vi "value to ring (portSpeed).vi"(11 "value":string) -> (3 "portSpeed":u32)   [LabVIEW 2020, in "AIM ARINC 664 Import.lvlib"]
uses:
  AIM ARINC 664 Import.lvlib
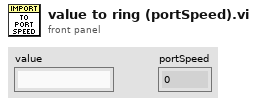
[diagram p1: front panel]
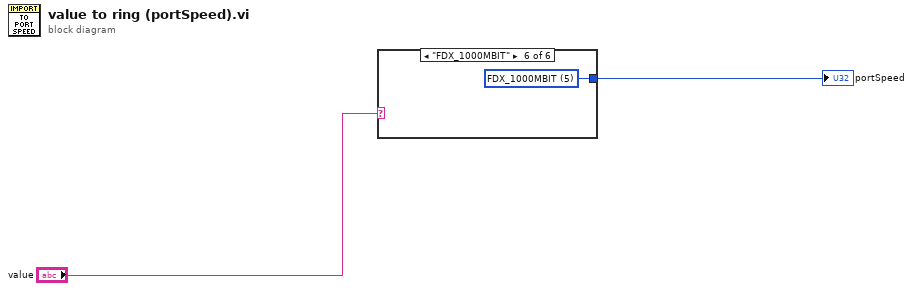
[diagram p0: block diagram]
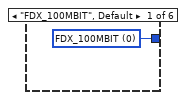
[diagram p2: hidden frame]
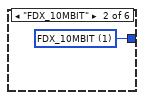
[diagram p3: hidden frame]
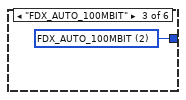
[diagram p4: hidden frame]
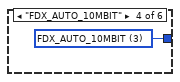
[diagram p5: hidden frame]
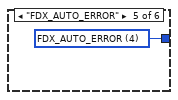
[diagram p6: hidden frame]
diagram:
  n1 = case shown="\"FDX_1000MBIT\"" "value" {
    tunnel: [w3 w4 w5 w6 w7 w8] -> w1
    frame "FDX_100MBIT", Default {
      w3 = u32 0 items=["FDX_100MBIT", "FDX_10MBIT", "FDX_AUTO_100MBIT", "FDX_AUTO_10MBIT", "FDX_AUTO_ERROR", "FDX_1000MBIT"] ("portSpeed")
    }
    frame "FDX_10MBIT" {
      w4 = u32 1 items=["FDX_100MBIT", "FDX_10MBIT", "FDX_AUTO_100MBIT", "FDX_AUTO_10MBIT", "FDX_AUTO_ERROR", "FDX_1000MBIT"] ("portSpeed")
    }
    frame "FDX_AUTO_100MBIT" {
      w5 = u32 2 items=["FDX_100MBIT", "FDX_10MBIT", "FDX_AUTO_100MBIT", "FDX_AUTO_10MBIT", "FDX_AUTO_ERROR", "FDX_1000MBIT"] ("portSpeed")
    }
    frame "FDX_AUTO_10MBIT" {
      w6 = u32 3 items=["FDX_100MBIT", "FDX_10MBIT", "FDX_AUTO_100MBIT", "FDX_AUTO_10MBIT", "FDX_AUTO_ERROR", "FDX_1000MBIT"] ("portSpeed")
    }
    frame "FDX_AUTO_ERROR" {
      w7 = u32 4 items=["FDX_100MBIT", "FDX_10MBIT", "FDX_AUTO_100MBIT", "FDX_AUTO_10MBIT", "FDX_AUTO_ERROR", "FDX_1000MBIT"] ("portSpeed")
    }
    frame "FDX_1000MBIT" {
      w8 = u32 5 items=["FDX_100MBIT", "FDX_10MBIT", "FDX_AUTO_100MBIT", "FDX_AUTO_10MBIT", "FDX_AUTO_ERROR", "FDX_1000MBIT"] ("portSpeed")
    }
  }
  "portSpeed" <- w1
